vi "Topmost VI Directory.vi"(4 "Relative path (.)":path=path "") -> (1 "Application Directory (+ Relative)":path)   [LabVIEW 2017]
doc: "Returns the directory of the top-level VI with Relative path (.) appended. In the development environment it falls back to the application directory."
uses:
  949d31c4-62ef-48f0-9511-4c05d3196e8d.vi
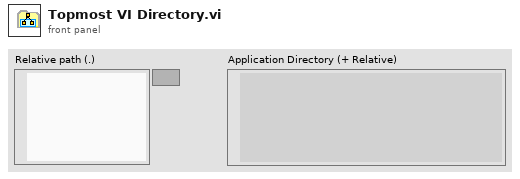
[diagram p1: front panel]
types:
  T1 = enum16{"Absolute path", "Relative path", "<Not A Path>"}
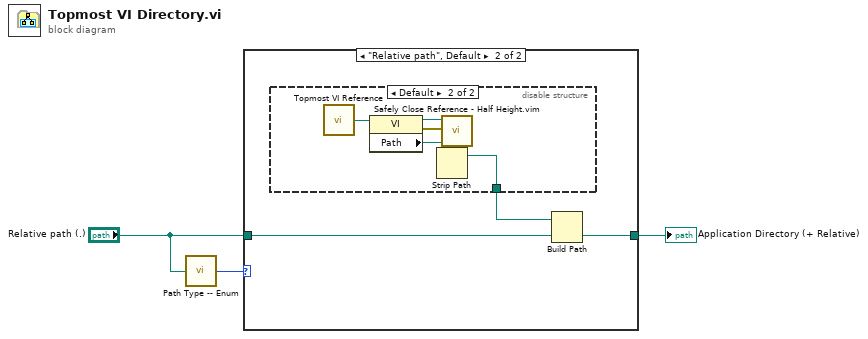
[diagram p0: block diagram]
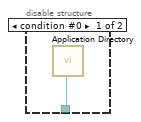
[diagram p3: hidden frame]
diagram:
  n1 = call "Path Type -- Enum.vi"("Value"="Relative path (.)") -> ("Enum"=w1:T1)
  n2 = case shown="\"Relative path\", Default" w1 {
    tunnel: [w4 w7] -> w3
    tunnel: "Relative path (.)" -> [w4 w5]
    frame "Absolute path" {
    }
    frame "Relative path", Default {
      n3 = disable-structure shown="Default" {
        disable-tunnel: [w8 w11] -> w6
        frame condition #0 {
          n4 = call <vilib>:"Application Directory.vi"() -> ("Application Directory"=w8:path)
        }
        frame condition #1 (active) {
          n5 = call "Topmost VI Reference.vi"() -> ("Topmost VI's Reference"=w12:refnum<vi>)  [unwired: 5 in]
          n6 = property class="VI"(reference=w12) -> (reference out=w10:refnum<vi>, error out=w9:errorcluster, "Path"=w13:path)  [unwired: 1 in]
          n7 = Strip Path(path=w13) -> (stripped path=w11:path)  [unwired: 1 out]
          n8 = call "Safely Close Reference - Half Height.vim"("error in (no error)"=w9, "Reference"=w10) -> ()  [unwired: 9 in, 1 out]
        }
      }
      n9 = Build Path(base path=w6, name or relative path=w5) -> (appended path=w7:path)
    }
  }
  "Application Directory (+ Relative)" <- w3
